vi "Send Log Status.vi"(8 "error in (no error)":errorcluster, 10 "String":string, 11 "Message Enqueuer in":refnum<class "Message Enqueuer.lvclass">) -> (0 "error out":errorcluster, 3 "Message Enqueuer out":refnum<class "Message Enqueuer.lvclass">)   [LabVIEW 2016, in "Controller Actor.lvlib" / "Log Status.lvclass"]
uses:
  <userlib>/Common Components/Controller/Messages/Log Status/Log Status.lvclass
  <vilib>/ActorFramework/Message Enqueuer/Message Enqueuer.lvclass
  C:/Program Files (x86)/National Instruments/LabVIEW 2016/vi.lib/ActorFramework/Message/Message.lvclass
  <vilib>/ActorFramework/Message Enqueuer/Message Enqueuer.lvclass/Message Enqueuer.ctl
  <vilib>/ActorFramework/Message Priority Queue/Priority Enqueue.vi
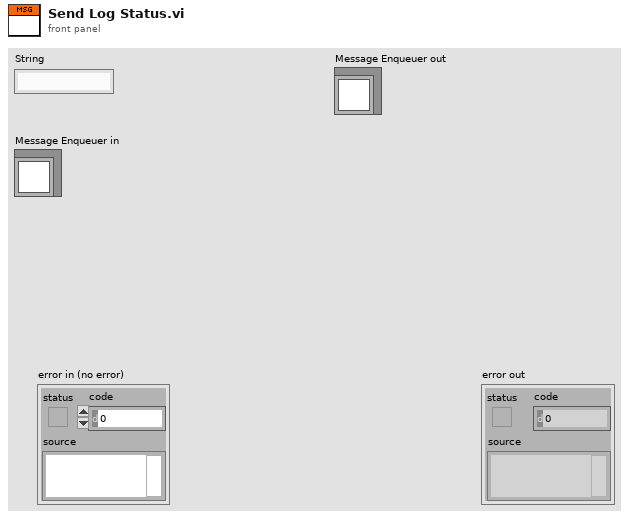
[diagram p1: front panel]
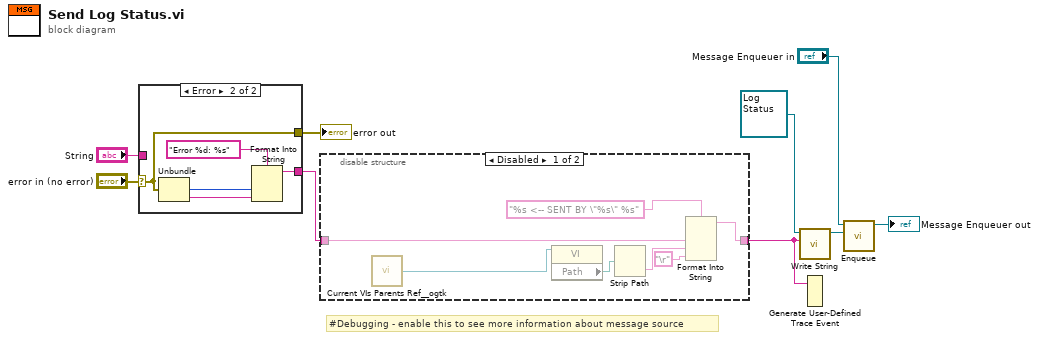
[diagram p0: block diagram]
diagram:
  # "#Debugging - enable this to see more information about message source"
  n1 = case shown="Error" "error in (no error)" {
    selector: "error in (no error)" -> [w11 w15]
    tunnel: [w11 w15] -> w4
    tunnel: [w10 w14] -> w2
    tunnel: "String" -> [w10 _]
    frame No Error {
    }
    frame Error {
      n2 = Unbundle(w15) -> ("code"=w12:i32, "source"=w13:string)  [unwired: 1 out]
      n3 = Format Into String(format string="Error %d: %s" ("String"), w12, w13) -> (resulting string=w14:string)  [unwired: 2 in, 1 out]
    }
  }
  "error out" <- w4
  n4 = disable-structure shown="Disabled" {
    disable-tunnel: w2 -> [w21 w24]
    disable-tunnel: [w20 w24] -> w1
    frame Disabled {
      n5 = call <userlib>:"Current VIs Parents Ref__ogtk.vi"() -> ("Calling VI's Reference"=w23:refnum<vi>)  [unwired: 2 in]
      n6 = property class="VI"(reference=w23) -> ("Path"=w18:path)  [unwired: 1 in, 2 out]
      n7 = Strip Path(path=w18) -> (name=w17:string)  [unwired: 1 out]
      n8 = Format Into String(format string="%s <-- SENT BY \"%s\" %s", w21, w17, "\r") -> (resulting string=w20:string)  [unwired: 2 in, 1 out]
    }
    frame Enabled {
    }
  }
  n9 = call <userlib>:"Write String.vi"("String"=w1, "Log Status in"=refnum<class "Log Status.lvclass"> refnum ("Log Status.lvclass")) -> ("Log Status out"=w8:refnum<class "Log Status.lvclass">)  [unwired: 8 in, 1 out]
  n10 = Generate User-Defined Trace Event(2:w1) -> ()  [unwired: 1 in]
  n11 = call <vilib>:"Enqueue.vi"("Message"=w8, "Message Enqueuer in"="Message Enqueuer in") -> ("Message Enqueuer out"=→"Message Enqueuer out":refnum<class "Message Enqueuer.lvclass">)  [unwired: 8 in, 1 out]
